vi "LiveSignal.vi"() -> ()   [LabVIEW 2022 SP3]
uses:
  ViolinSubs/PreferencesControl.ctl
  <extravilib>/ChannelInstances/Lossy Stream-a[.](wfm(dbl))/EndpointRead.vi
  ViolinSubs/Mic/Mic_Global.vi
  <extravilib>/ChannelInstances/Tag-a[.](wfm(dbl))/Instantiate.vi
  <extravilib>/ChannelInstances/Lossy Stream-a[.](wfm(dbl))/Instantiate.vi
  <extravilib>/ChannelInstances/Lossy Stream-a[.](wfm(dbl))/)Channel.vi
  <resource>/ChannelSupport/_ChannelSupport/WaitIfNeeded.vi
  <extravilib>/ChannelInstances/Tag-a[.](wfm(dbl))/EndpointRead.vi
  <extravilib>/ChannelInstances/Tag-a[.](wfm(dbl)).lvlib
  <extravilib>/ChannelInstances/Lossy Stream-a[.](wfm(dbl)).lvlib
  <vilib>/Analysis/NI_AALPro.lvlib
panel:
  in  "Load a Template":bool
  in  "autoscale":bool
  in  "Save as a Template":bool
  in  "device:":u16(ring) items=["BuerginBase Microphone", "485B39 200083408035100798118210422", "MacBook Pro Microphone", "Camo Microphone", "Microsoft Teams Audio", "ZoomAudioDevice"]
  out "data":waveform(dbl)[](array[waveform])
  in  "Tab Control":T1(tab)
  in  "Magnitude Averages":u8(slide)=25 scale=1.0..50.0
  out "Hammer":waveform(dbl)(graph)
  out "Microphone":waveform(dbl)(graph)
  out "Power Spectrum":waveform(dbl)(graph)
  out "Cal Hammer":waveform(dbl)[](graph)
  out "cal Mic":waveform(dbl)[](graph)
  out "Power Spectrum 2":waveform(dbl)(graph)
  in  "In->Out":bool
  in  "Out->In":bool
  out "Trig Mic":waveform(dbl)[](graph)
  out "Trig Hammer":waveform(dbl)[](graph)
  out "Triggered Spectrum":waveform(dbl)(graph)
  out "Real/Imag":cluster{dbl, "df":dbl, dbl[]}[](graph)
  out "Average FRF":cluster{dbl, "df":dbl, dbl[]}(graph)
  in  "Offset (msec)":dbl(slide) scale=0.0..10.0
  in  "Settings":T2={"Name of test"="", "Date"=timestamp(0 s since 1904-01-01), "Location"="", "Template"="", "Soundcard"="", "resolution"=32, "Sampling rate"=48000, "Ch1 Gain "=0.0, "Ch2 Gain"=0.0, "Sample time (s)"=0.3, "Pre-trigger (s)"=0.01, "Hammer Threshold"=0.01, "Positions"=12, "Taps/Position"=5, "Set Names"="", "Freq resolution"=1.0, "Hammer cutoff"=1.0, "Mic cutoff"=1.0, "Double bounce "=0.0, "Hammer Cal"=1.0, "dB Offset"=0.0, "Accel Cal"=10.0, "Vibrometer Cal"=0.0, "Mic Cal"=1.0, "Output"=2, "Voltage Cal"=1.0, "Vibrometer Port"="ASRL27::INSTR", "Range"=10, "High Pass"=2, "Bandwidth"=25, "X Range"=[], "Y Range"=[], "dB Spread"=40.0, "Trigger"=0, "Ch_1"=1, "Ch_2"=2, "flip?"=FALSE, "60Hz"=FALSE, "Time offset"=0.0, "Piezo Cal"=1.0, "Default Notes"=""} {"Ch_2" min=1 step=1; "Ch_1" min=1 max=100 step=1; "Trigger" items=["Hammer (force)", "Self-tap", "Spacebar"]; "Bandwidth" items=["1 kHz"=1, "5 kHz"=5, "10 kHz"=10, "25 kHz"=25, "50 kHz"=50, "100 kHz"=100]; "High Pass" items=["Off", "13 Hz", "104 Hz"]; "Range" items=["10 mm/s"=1, "20 mm/s"=2, "50 mm/s"=5, "100 mm/s"=10, "200 mm/s"=20, "500 mm/s"=50, "1 m/s"=100, "2 m/s"=200]; "Output" items=["Accelerometer", "Speed (from acceleration)", "Microphone", "Vibrometer", "Piezo"]; "Voltage Cal" format="%#_13g"; "Ch2 Gain" format="%#_13g"; "Ch1 Gain" format="%#_13g"; "Double bounce" min=0.0; "Mic cutoff" min=0.0 format="%#_4g"; "Hammer cutoff" min=0.0 format="%#_4g"; "Freq resolution" min=0.0; "Pre-trigger (s)" format="%#_13g"; "Date" format="%<%H:%M\n%d/%m/%y>T"; "resolution" items=["16 bit"=16, "24 bit"=24, "32 bit"=32]; "Sampling rate" items=["22050 samp/s"=22050, "44100 samp/s"=44100, "48000 samp/s"=48000]}
  # "For Mac mic - start running and then have both channels on 1"
  # "Raw values from the Soundcard"
  # "Calibrated Values"
  # "All values are calibrated, arrows sync x axes"
  # "Hz"
  # "dB"
  # "dB"
  # "sec"
  # "sec"
  # "mV/Pa"
  # "mV/m/s2"
  # "mV/mm/s"
  # "V/N"
  # "sec"
  # "sec"
  # "mV/N"
  # "a.u."
  # "a.u."
  # "sec"
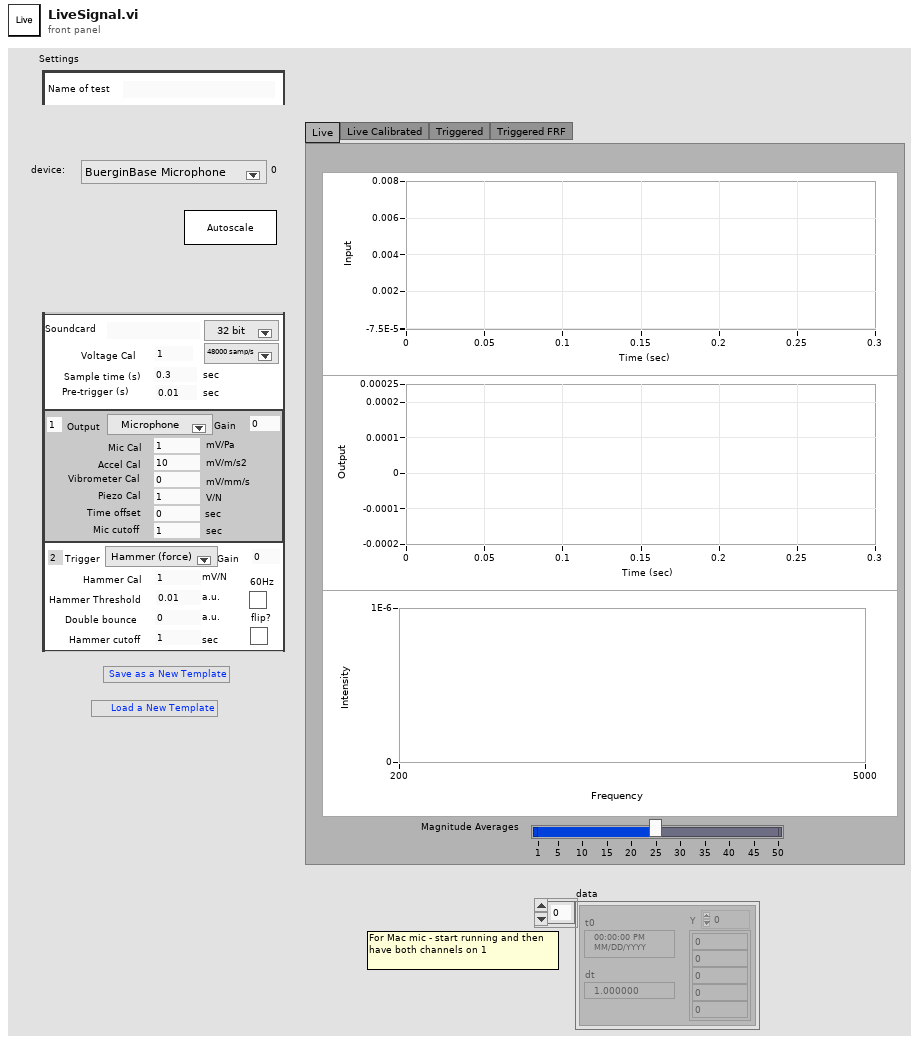
[diagram p1: front panel]
types:
  T1 = enum32{"Live", "Live Calibrated", "Triggered", "Triggered FRF"}
  T2 = typedef "PreferencesControl.ctl" = cluster{"Name of test":string, "Date":timestamp, "Location":string, "Template":string, "Soundcard":string, "resolution":u16, "Sampling rate":u16, "Ch1 Gain ":dbl, "Ch2 Gain":dbl, "Sample time (s)":dbl, "Pre-trigger (s)":dbl, "Hammer Threshold":dbl, "Positions":i16, "Taps/Position":i16, "Set Names":string, "Freq resolution":dbl, "Hammer cutoff":dbl, "Mic cutoff":dbl, "Double bounce ":dbl, "Hammer Cal":dbl, "dB Offset":dbl, "Accel Cal":dbl, "Vibrometer Cal":dbl, "Mic Cal":dbl, "Output":u16, "Voltage Cal":dbl, "Vibrometer Port":refnum<visa-resource-name>, "Range":u16, "High Pass":u16, "Bandwidth":u16, "X Range":cluster{"Minimum":dbl, "Maximum":dbl, "Increment":dbl, "Minor Increment":dbl, "Start":dbl}[], "Y Range":cluster{"Minimum":dbl, "Maximum":dbl, "Increment":dbl, "Minor Increment":dbl, "Start":dbl}[], "dB Spread":dbl, "Trigger":u16, "Ch_1":u8, "Ch_2":u8, "flip?":bool, "60Hz":bool, "Time offset":dbl, "Piezo Cal":dbl, "Default Notes":string}
  T3 = typedef "Tag-a[.](wfm(dbl)).lvlib/))Channel.ctl" = refnum<queue>
  T4 = typedef "Lossy Stream-a[.](wfm(dbl)).lvlib/)Channel.ctl" = refnum<queue>
  T5 = enum8{"Enabled", "Disabled", "Disabled and Grayed Out"}
  T6 = typedef "LVRangeTypeDef.ctl" = cluster{"Minimum":dbl, "Maximum":dbl, "Increment":dbl, "Minor Increment":dbl, "Start":dbl}
  T7 = enum16{"Initialize", "Free run", "One Shot - waiting", "One Shot - triggered", "Wait", "Close"}
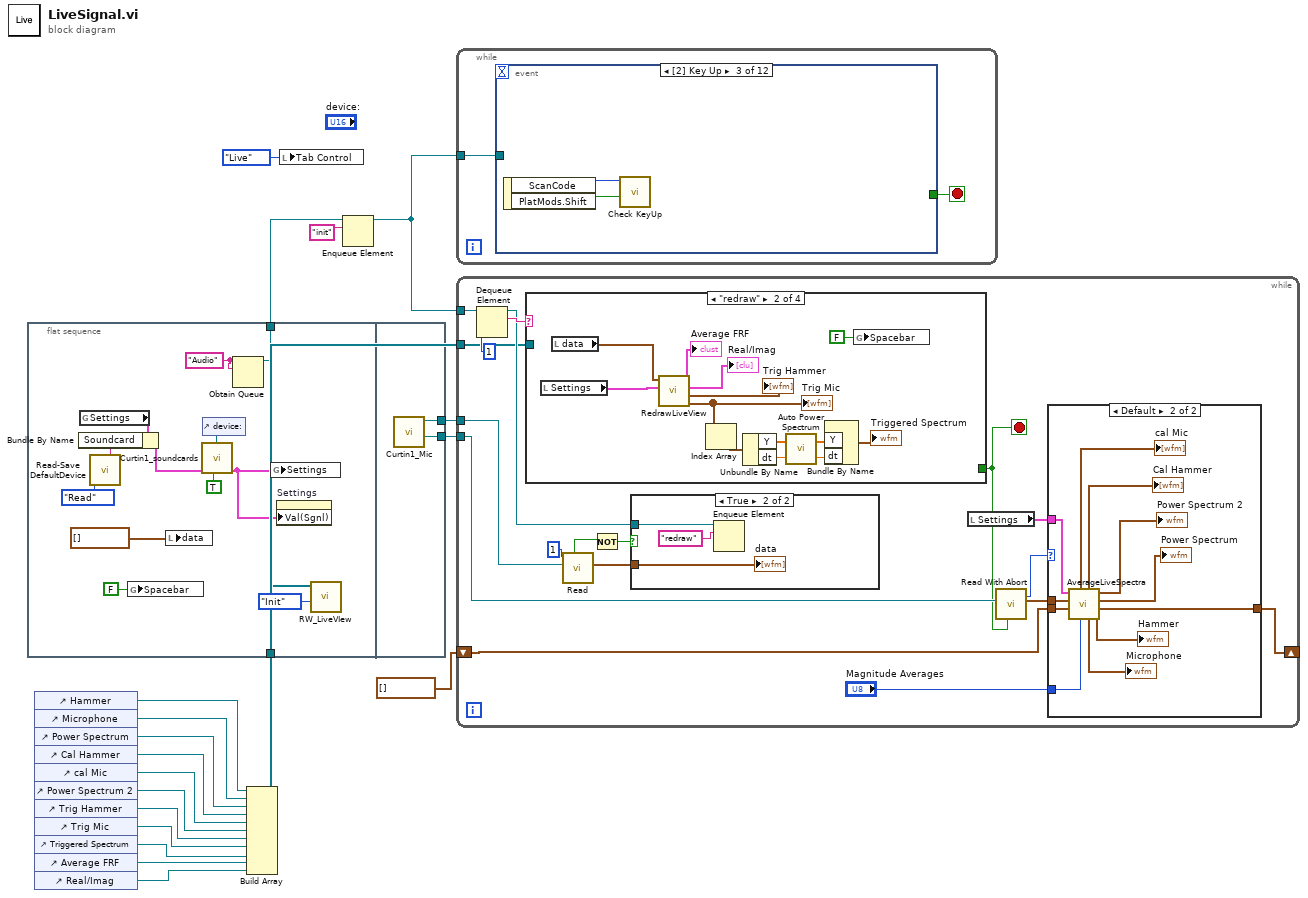
[diagram p0: block diagram]
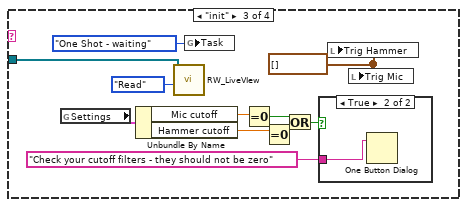
[diagram p5: hidden frame]
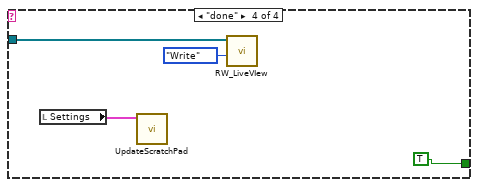
[diagram p7: hidden frame]
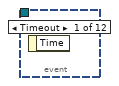
[diagram p8: hidden frame]
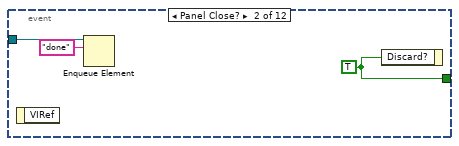
[diagram p9: hidden frame]
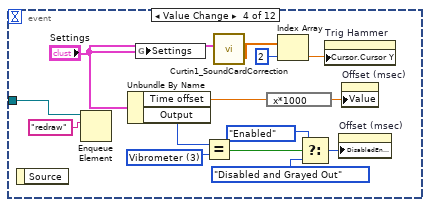
[diagram p10: hidden frame]
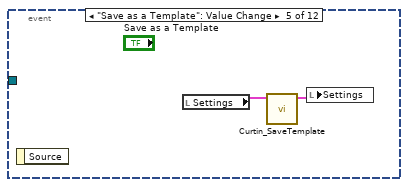
[diagram p11: hidden frame]
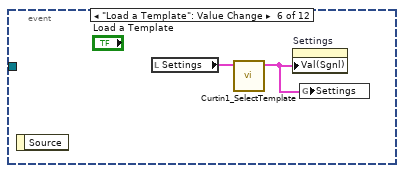
[diagram p12: hidden frame]
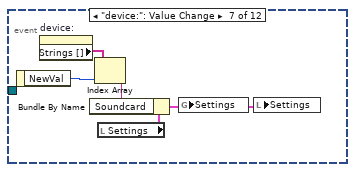
[diagram p13: hidden frame]
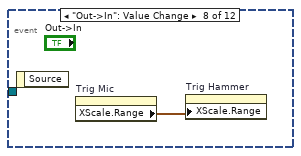
[diagram p14: hidden frame]
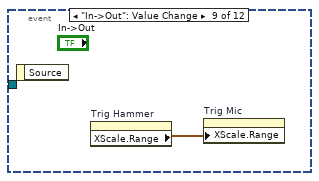
[diagram p15: hidden frame]
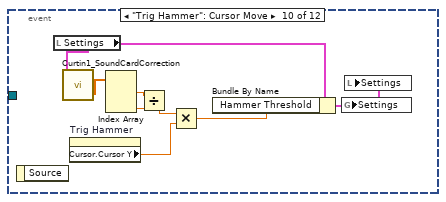
[diagram p16: hidden frame]
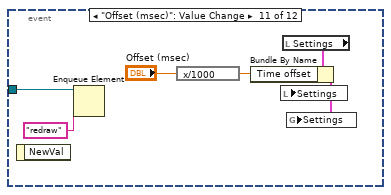
[diagram p17: hidden frame]
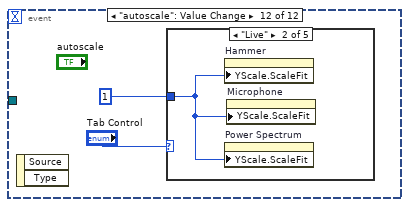
[diagram p18: hidden frame]
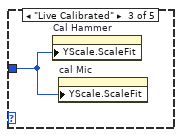
[diagram p20: hidden frame]
diagram:
  n1 = flat-sequence {
    tunnel: [w26] -> w15
    tunnel: w2 -> [w22]
    tunnel: [w34] -> w19
    tunnel: [w33] -> w18
    frame #0 {
      w27 = "Audio" ("name (unnamed)")
      n2 = global read "Mic_Global.vi" "Settings"() -> (w30:T2)
      n3 = call "Read-Save DefaultDevice.vi"("Task"=enum16{"Save", "Read"}."Read") -> ("Soundcard Out"=w29:string)  [unwired: 9 in, 1 out]
      n4 = Bundle By Name(cluster=w30, "Soundcard"=w29) -> (w25:T2)
      n5 = global write "Mic_Global.vi" "Spacebar"(FALSE ("Spacebar")) -> ()
      n6 = local write "data"(waveform(dbl)[] [] ("data")) -> ()
      n7 = control-ref of="device:"() -> (w32:refnum<vi>)
      n8 = call "Curtin1_soundcards.vi"("hush?"=TRUE, "Settings In"=w25, "device:"=w32) -> ("Settings Out"=w24:T2)  [unwired: 7 in, 1 out]
      n9 = Obtain Queue(name (unnamed)=w27, element data type=w27) -> (queue out=w26:refnum<queue>)  [unwired: 3 in, 2 out]
      n10 = global write "Mic_Global.vi" "Settings"(w24) -> ()
      n11 = property on="Settings" class="Clust (strict)"("Val(Sgnl)"=w24) -> ()  [unwired: 2 in, 2 out]
      n12 = call "RW_LiveVIew.vi"("Task"=enum16{"Read", "Write", "Init"}."Init", "Plots"=w22) -> ()  [unwired: 10 in]
    }
    frame #1 {
      n13 = call "Curtin1_Mic.vi"() -> ("latest data"=w33:T3, "Tap"=w34:T4)  [unwired: 10 in]
    }
  }
  n14 = control-ref of="Hammer"() -> (w13:refnum<vi>)
  n15 = control-ref of="Microphone"() -> (w12:refnum<vi>)
  n16 = control-ref of="Power Spectrum"() -> (w11:refnum<vi>)
  n17 = control-ref of="Cal Hammer"() -> (w10:refnum<vi>)
  n18 = control-ref of="cal Mic"() -> (w9:refnum<vi>)
  n19 = control-ref of="Power Spectrum 2"() -> (w8:refnum<vi>)
  n20 = control-ref of="Trig Hammer"() -> (w7:refnum<vi>)
  n21 = control-ref of="Trig Mic"() -> (w6:refnum<vi>)
  n22 = control-ref of="Triggered Spectrum"() -> (w5:refnum<vi>)
  n23 = control-ref of="Average FRF"() -> (w4:refnum<vi>)
  n24 = control-ref of="Real/Imag"() -> (w3:refnum<vi>)
  n25 = Build Array(w13, w12, w11, w10, w9, w8, w7, w6, w5, w4, w3) -> (w2:refnum<vi>[])
  n26 = local write "Tab Control"(T1."Live" ("Tab Control")) -> ()
  n27 = Enqueue Element(queue=w15, element="init") -> (queue out=w16:refnum<queue>)  [unwired: 2 in, 2 out]
  n28 = while {
    tunnel: w16 -> [w36]
    stop <- w35 stop-if-true
    n29 = event shown="[2] Key Up" {
      selector: _ -> [_ _ _ _ _ _ _ _ _ _ _ _]
      dyn-events: _ -> [_ _ _ _ _ _ _ _ _ _ _ _]
      timeout: _ -> [_ _ _ _ _ _ _ _ _ _ _ _]
      tunnel: [_ w39 _ _ _ _ _ _ _ _ _ _] -> w35
      tunnel: w36 -> [_ w38 _ w54 _ _ _ _ _ _ w75 _]
      event Timeout {
        n30 = event-data() -> ()  [unwired: 1 in, 1 out]
      }
      event Panel Close? {
        w39 = TRUE ("Discard?")
        n31 = event-data() -> ()  [unwired: 1 in, 1 out]
        n32 = Enqueue Element(queue=w38, element="done") -> ()  [unwired: 2 in, 3 out]
        n33 = event-data("Discard?"=w39) -> ()  [unwired: 1 in, 1 out]
      }
      event Key Up {
        n34 = event-data() -> ("ScanCode"=w41:i16, "PlatMods.Shift"=w40:bool)  [unwired: 1 in]
        n35 = call "Check KeyUp.vi"("Shift"=w40, "ScanCode"=w41) -> ()  [unwired: 9 in, 1 out]
      }
      event Value Change {
        w43 = u16 3 items=["Accelerometer", "Accel (speed)", "Microphone", "Vibrometer"] ("Output")
        n36 = event-data() -> ()  [unwired: 1 in, 1 out]
        n37 = Enqueue Element(queue=w54, element="redraw") -> ()  [unwired: 2 in, 3 out]
        n38 = Unbundle By Name("Settings") -> ("Time offset"=w53:dbl, "Output"=w44:u16)
        n39 = global write "Mic_Global.vi" "Settings"("Settings") -> ()
        n40 = Equal?(x=w44, y=w43) -> (x = y?=w45:bool)
        n41 = call "Curtin1_SoundCardCorrection.vi"("Settings"="Settings") -> ("Converted"=w50:dbl[])  [unwired: 5 in, 5 out]
        n42 = expression code="x*1000"(w53) -> (w52:dbl)
        n43 = Index Array(array=w50, index=2) -> (element=w48:dbl)
        n44 = Select(t=T5."Enabled" ("Disabled"), s=w45, f=T5."Disabled and Grayed Out" ("Disabled")) -> (s? t:f=w47:T5)
        n45 = property on="Trig Hammer" class="WFGraph (strict)"("Cursor.Cursor Y"=w48) -> ()  [unwired: 2 in, 2 out]
        n46 = property on="Offset (msec)" class="Slide (strict)"("DisabledEnum"=w47) -> ()  [unwired: 2 in, 2 out]
        n47 = property on="Offset (msec)" class="Slide (strict)"("Value"=w52) -> ()  [unwired: 2 in, 2 out]
      }
      event "Save as a Template": Value Change {
        n48 = event-data() -> ()  [unwired: 1 in, 1 out]
        n49 = local read "Settings"() -> (w57:T2)
        n50 = call "Curtin_SaveTemplate.vi"("Settings in"=w57) -> ("Settings out"=w56:T2)  [unwired: 8 in, 2 out]
        n51 = local write "Settings"(w56) -> ()
      }
      event "Load a Template": Value Change {
        n52 = event-data() -> ()  [unwired: 1 in, 1 out]
        n53 = local read "Settings"() -> (w59:T2)
        n54 = call "Curtin1_SelectTemplate.vi"("Settings in"=w59) -> ("Settings out"=w58:T2)  [unwired: 9 in, 1 out]
        n55 = property on="Settings" class="Clust (strict)"("Val(Sgnl)"=w58) -> ()  [unwired: 2 in, 2 out]
        n56 = global write "Mic_Global.vi" "Settings"(w58) -> ()
      }
      event "device:": Value Change {
        n57 = event-data() -> ("NewVal"=w63:u16)  [unwired: 1 in]
        n58 = property on="device:" class="Ring (strict)"() -> ("Strings []"=w64:string[])  [unwired: 2 in, 2 out]
        n59 = Index Array(array=w64, index=w63) -> (element=w61:string)
        n60 = local read "Settings"() -> (w62:T2)
        n61 = Bundle By Name(cluster=w62, "Soundcard"=w61) -> (w60:T2)
        n62 = global write "Mic_Global.vi" "Settings"(w60) -> ()
        n63 = local write "Settings"(w60) -> ()
      }
      event "Out->In": Value Change {
        n64 = event-data() -> ()  [unwired: 1 in, 1 out]
        n65 = property on="Trig Mic" class="WFGraph (strict)"() -> ("XScale.Range"=w65:T6)  [unwired: 2 in, 2 out]
        n66 = property on="Trig Hammer" class="WFGraph (strict)"("XScale.Range"=w65) -> ()  [unwired: 2 in, 2 out]
      }
      event "In->Out": Value Change {
        n67 = event-data() -> ()  [unwired: 1 in, 1 out]
        n68 = property on="Trig Hammer" class="WFGraph (strict)"() -> ("XScale.Range"=w66:T6)  [unwired: 2 in, 2 out]
        n69 = property on="Trig Mic" class="WFGraph (strict)"("XScale.Range"=w66) -> ()  [unwired: 2 in, 2 out]
      }
      event "Trig Hammer": Cursor Move {
        n70 = event-data() -> ()  [unwired: 1 in, 1 out]
        n71 = local read "Settings"() -> (w67:T2)
        n72 = call "Curtin1_SoundCardCorrection.vi"("Settings"=w67) -> ("Converted"=w73:dbl[])  [unwired: 5 in, 5 out]
        n73 = property on="Trig Hammer" class="WFGraph (strict)"() -> ("Cursor.Cursor Y"=w69:dbl)  [unwired: 2 in, 2 out]
        n74 = Index Array(array=w73) -> (element #1=w72:dbl, element #3=w71:dbl)  [unwired: 3 in, 1 out]
        n75 = Divide(x=w72, y=w71) -> (x/y=w70:dbl)
        n76 = Multiply(x=w70, y=w69) -> (x*y=w68:dbl)
        n77 = Bundle By Name(cluster=w67, "Hammer Threshold"=w68) -> (w74:T2)
        n78 = global write "Mic_Global.vi" "Settings"(w74) -> ()
        n79 = local write "Settings"(w74) -> ()
      }
      event "Offset (msec)": Value Change {
        n80 = event-data() -> ()  [unwired: 1 in, 1 out]
        n81 = Enqueue Element(queue=w75, element="redraw") -> ()  [unwired: 2 in, 3 out]
        n82 = expression code="x/1000"("Offset (msec)") -> (w77:dbl)
        n83 = local read "Settings"() -> (w80:T2)
        n84 = Bundle By Name(cluster=w80, "Time offset"=w77) -> (w79:T2)
        n85 = local write "Settings"(w79) -> ()
        n86 = global write "Mic_Global.vi" "Settings"(w79) -> ()
      }
      event "autoscale": Value Change {
        n87 = event-data() -> ()  [unwired: 1 in, 2 out]
        n88 = case shown="\"Live\"" "Tab Control" {
          tunnel: u8 1 ("Y Scale.Scale Fit") -> [_ w83 w84 w85 w86]
          frame Default {
          }
          frame "Live" {
            n89 = property on="Hammer" class="WFGraph (strict)"("YScale.ScaleFit"=w83) -> ()  [unwired: 2 in, 2 out]
            n90 = property on="Power Spectrum" class="WFGraph (strict)"("YScale.ScaleFit"=w83) -> ()  [unwired: 2 in, 2 out]
            n91 = property on="Microphone" class="WFGraph (strict)"("YScale.ScaleFit"=w83) -> ()  [unwired: 2 in, 2 out]
          }
          frame "Live Calibrated" {
            n92 = property on="Cal Hammer" class="WFGraph (strict)"("YScale.ScaleFit"=w84) -> ()  [unwired: 2 in, 2 out]
            n93 = property on="cal Mic" class="WFGraph (strict)"("YScale.ScaleFit"=w84) -> ()  [unwired: 2 in, 2 out]
          }
          frame "Triggered" {
            n94 = property on="Trig Hammer" class="WFGraph (strict)"("YScale.ScaleFit"=w85) -> ()  [unwired: 2 in, 2 out]
            n95 = property on="Trig Mic" class="WFGraph (strict)"("YScale.ScaleFit"=w85) -> ()  [unwired: 2 in, 2 out]
            n96 = property on="Triggered Spectrum" class="WFGraph (strict)"("YScale.ScaleFit"=w85) -> ()  [unwired: 2 in, 2 out]
          }
          frame "Triggered FRF" {
            n97 = property on="Real/Imag" class="WFGraph (strict)"("YScale.ScaleFit"=w86) -> ()  [unwired: 2 in, 2 out]
            n98 = property on="Average FRF" class="WFGraph (strict)"("YScale.ScaleFit"=w86) -> ()  [unwired: 2 in, 2 out]
          }
        }
      }
    }
  }
  n99 = while {
    tunnel: w16 -> [w104]
    tunnel: w19 -> [w96]
    tunnel: w18 -> [w101]
    tunnel: w2 -> [w92]
    shift-right: [w89] -> _
    shift-left: waveform(dbl)[] [] -> [w91]
    stop <- w100 stop-if-true
    n100 = Dequeue Element(queue=w104, timeout in ms (-1)=1) -> (queue out=w94:refnum<queue>, element=w103:string)  [unwired: 1 in, 2 out]
    n101 = case shown="\"redraw\"" w103 {
      tunnel: [_ _ _ TRUE ("Discard?")] -> w100
      tunnel: w92 -> [_ _ w133 w145]
      frame Default {
      }
      frame "redraw" {
        n102 = local read "Settings"() -> (w131:T2)
        n103 = local read "data"() -> (w132:waveform(dbl)[])
        n104 = call "RedrawLiveView.vi"("Settings"=w131, "data"=w132) -> ("Trig Mic"=w123:waveform(dbl)[], "Trig Hammer"=→"Trig Hammer":waveform(dbl)[], "Real/Imag"=→"Real/Imag":cluster{dbl, "df":dbl, dbl[]}[], "Average FRF"=→"Average FRF":cluster{dbl, "df":dbl, dbl[]})  [unwired: 6 in]
        "Trig Mic" <- w123
        n105 = Index Array(array=w123) -> (element=w122:waveform(dbl))  [unwired: 1 in]
        n106 = Unbundle By Name(w122) -> ("Y"=w127:dbl[], "dt"=w126:dbl)
        n107 = call <vilib>:"Auto Power Spectrum.vi"("dt"=w126, "Signal (V)"=w127) -> ("df"=w124:dbl, "Power Spectrum (V^2 rms)"=w125:dbl[])
        n108 = Bundle By Name("Y"=w125, "dt"=w124) -> (→"Triggered Spectrum":waveform(dbl))  [unwired: 1 in]
        n109 = global write "Mic_Global.vi" "Spacebar"(FALSE ("Spacebar")) -> ()
      }
      frame "init" {
        w142 = waveform(dbl)[] [] ("Hammer 2")
        n110 = global read "Mic_Global.vi" "Settings"() -> (w141:T2)
        n111 = Unbundle By Name(w141) -> ("Mic cutoff"=w140:dbl, "Hammer cutoff"=w139:dbl)
        n112 = call "RW_LiveVIew.vi"("Task"=enum16{"Read", "Write", "Init"}."Read", "Plots"=w133) -> ()  [unwired: 10 in]
        n113 = global write "Mic_Global.vi" "Task"(T7."One Shot - waiting" ("Task")) -> ()
        n114 = Equal To 0?(x=w140) -> (x = 0?=w138:bool)
        n115 = Equal To 0?(x=w139) -> (x = 0?=w137:bool)
        n116 = Or(x=w138, y=w137) -> (x .or. y?=w135:bool)
        n117 = case shown="True" w135 {
          tunnel: "Check your cutoff filters - they should not be zero" ("element") -> [_ w144]
          frame False {
          }
          frame True {
            n118 = One Button Dialog(message=w144) -> ()  [unwired: 1 in, 1 out]
          }
        }
        n119 = local write "Trig Hammer"(w142) -> ()
        n120 = local write "Trig Mic"(w142) -> ()
      }
      frame "done" {
        n121 = local read "Settings"() -> (w147:T2)
        n122 = call "UpdateScratchPad.vi"("Settings"=w147) -> ()  [unwired: 9 in, 2 out]
        n123 = call "RW_LiveVIew.vi"("Task"=enum16{"Read", "Write", "Init"}."Write", "Plots"=w145) -> ()  [unwired: 10 in]
      }
    }
    n124 = call <extravilib>:"Read.vi"("channel"=w96, "timeout in ms (-1)"=1) -> ("element"=w99:waveform(dbl)[], "timed out?"=w98:bool)  [unwired: 4 in, 4 out]
    n125 = Not(x=w98) -> (.not. x?=w97:bool)
    n126 = case shown="True" w97 {
      tunnel: w99 -> [_ w119]
      tunnel: w94 -> [_ w117]
      frame False {
      }
      frame True {
        n127 = Enqueue Element(queue=w117, element="redraw") -> ()  [unwired: 2 in, 3 out]
        "data" <- w119
      }
    }
    n128 = local read "Settings"() -> (w93:T2)
    n129 = call <extravilib>:"Read With Abort.vi"("abort"=w100, "channel"=w101) -> ("element"=w88:waveform(dbl)[], "missed"=w87:i32)  [unwired: 7 in, 1 out]
    n130 = case shown="Default" w87 {
      tunnel: w93 -> [_ w116]
      tunnel: w88 -> [_ w115]
      tunnel: w91 -> [w105 w114]
      tunnel: "Magnitude Averages" -> [_ w113]
      tunnel: [w105 w106] -> w89
      frame -1 {
      }
      frame Default {
        n131 = call "AverageLiveSpectra.vi"("Magnitude Averages"=w113, "old reading"=w114, "new reading"=w115, "Settings"=w116) -> ("Hammer"=→"Hammer":waveform(dbl), "FIFO out"=w106:waveform(dbl)[], "average spectrum"=→"Power Spectrum":waveform(dbl), "Power Spectrum"=→"Power Spectrum 2":waveform(dbl), "Microphone"=→"Microphone":waveform(dbl), "Cal Hammer"=→"Cal Hammer":waveform(dbl)[], "cal Mic"=→"cal Mic":waveform(dbl)[])  [unwired: 1 in]
      }
    }
  }
